vi "ARRAY2D.vi"() -> ()   [LabVIEW 2014]
doc: "This function squares each value in the 2-D array.\n\nFor information on the data types used for the DLL function, right-click on the Call Library Function node and choose Configure."
uses:
  CLF_Example.dll
panel:
  out "output":dbl[][](array[numeric])
  in  "input":dbl[][](array[numeric])=[[0.0, 1.0], [2.0, 3.0], [4.0, 5.0], [6.0, 7.0]]
  # "See the block diagram for more information."
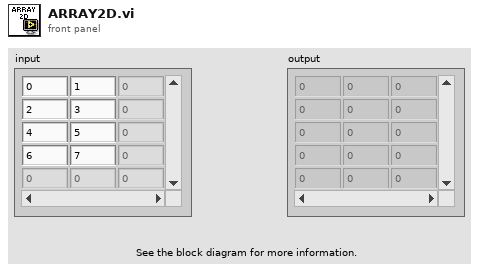
[diagram p1: front panel]
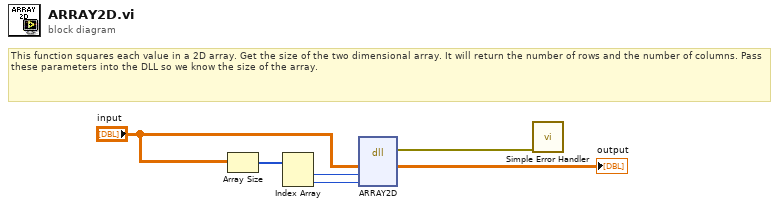
[diagram p0: block diagram]
diagram:
  # "This function squares each value in a 2D array. Get the size of the two dimensional array. It will return the number of rows and the number of columns. Pass these parameters into the DLL so we know the size of the array."
  n1 = Array Size(array="input") -> (size(s)=w4:i32[])
  n2 = Index Array(array=w4) -> (element #1=w3:i32, element #2=w2:i32)  [unwired: 2 in]
  n3 = dll-call lib="e:/builds/penguin/labview/branches/2014/dev/dist/examples/Connectivity/Libraries and Executables/DLL Calling VIs/CLF_Example**.*" fn="ARRAY2D"("array"="input", "array_length_row"=w3, "array_length_col"=w2) -> (error out=w1:errorcluster, "array"=→"output":dbl[][])  [unwired: 5 in, 2 out]
  n4 = call <vilib>:"Simple Error Handler.vi"("error in (no error)"=w1) -> ()  [unwired: 4 in, 5 out]
